vi "Write Loads.vi"(8 "error in (no error)":errorcluster, 10 "Loads":T1[](array[typedef]) {"PowerMax" items=["24 ", "48", "96"]; "Mode" min=0 max=12 step=1}, 11 "NhRegenGridSim in":refnum<class "NhRegenGridSim.lvclass">) -> (0 "error out":errorcluster, 3 "NhRegenGridSim out":refnum<class "NhRegenGridSim.lvclass">)   [LabVIEW 2018, in "AcPwrPlugins.lvlib" / "NhRegenGridSim.lvclass"]
uses:
  NhRegenGridSim.lvclass
  TypeDefs/Load.ctl
  TypeDefs/SlewRates.ctl
  TypeDefs/LoadSettings.ctl
  TypeDefs/Measurements.ctl
  TypeDefs/Ranges.ctl
  NhRegenGridSim.lvclass/NhRegenGridSim.ctl
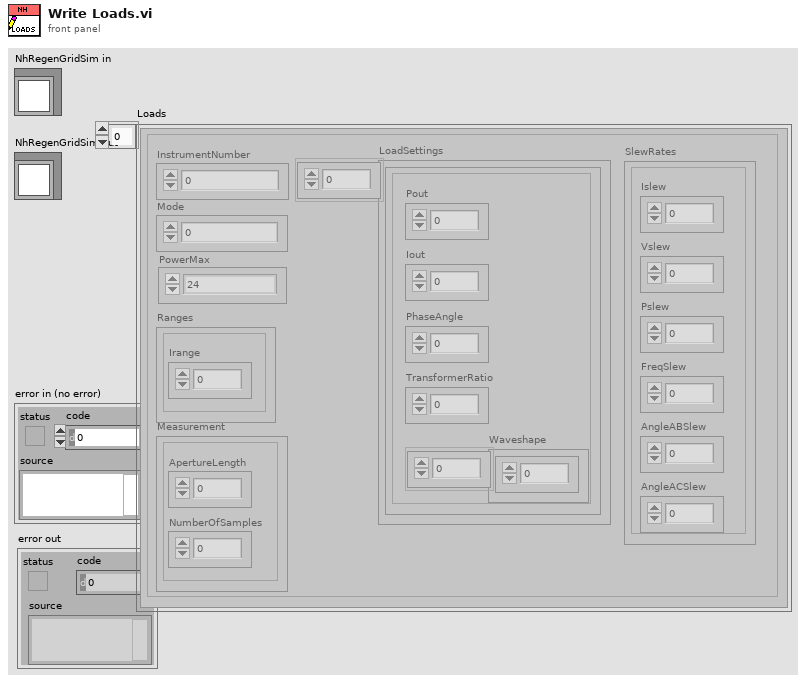
[diagram p1: front panel]
types:
  T1 = typedef "AcPwrPlugins.lvlib/NhRegenGridSim.lvclass/Load.ctl" = cluster{"SlewRates":T2, "LoadSettings":T3, "Measurement":T4, "Ranges":T5, "Mode":i32, "InstrumentNumber":u32, "PowerMax":u16}
  T2 = typedef "AcPwrPlugins.lvlib/NhRegenGridSim.lvclass/SlewRates.ctl" = cluster{"Islew":dbl, "Vslew":dbl, "Pslew":dbl, "FreqSlew":dbl, "AngleABSlew":dbl, "AngleACSlew":dbl}
  T3 = typedef "AcPwrPlugins.lvlib/NhRegenGridSim.lvclass/LoadSettings.ctl" = cluster{"Pout":dbl, "Iout":dbl, "PhaseAngle":dbl, "TransformerRatio":dbl, "Waveshape":dbl[]}[]
  T4 = typedef "AcPwrPlugins.lvlib/NhRegenGridSim.lvclass/Measurements.ctl" = cluster{"ApertureLength":dbl, "NumberOfSamples":u32}
  T5 = typedef "AcPwrPlugins.lvlib/NhRegenGridSim.lvclass/Ranges.ctl" = cluster{"Irange":dbl}
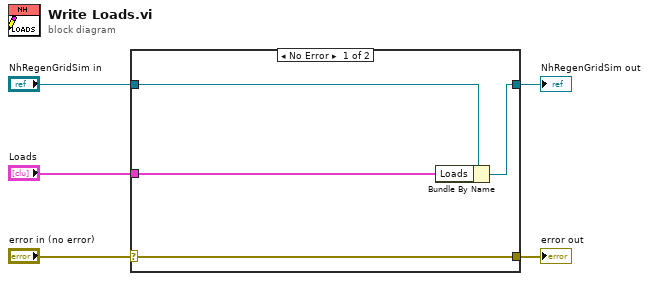
[diagram p0: block diagram]
diagram:
  n1 = case shown="No Error" "error in (no error)" {
    selector: "error in (no error)" -> [w9 w10]
    tunnel: [w9 w10] -> w4
    tunnel: [w7 w11] -> w2
    tunnel: "NhRegenGridSim in" -> [w8 w11]
    tunnel: "Loads" -> [w6 _]
    frame No Error {
      n2 = Bundle By Name(cluster=w8, "Loads"=w6) -> (w7:refnum<class "NhRegenGridSim.lvclass">)
    }
    frame Error {
    }
  }
  "error out" <- w4
  "NhRegenGridSim out" <- w2
